vi "FBProjectVI.vi"(11 "Element":dbl=8.0) -> (0 "Element Index":dbl=3.0, 3 "Element Found":bool=TRUE)   [LabVIEW 2023]
doc: "Array = {5,3,8,9,1}\nOutput = Index of element"
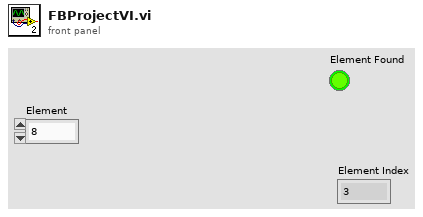
[diagram p1: front panel]
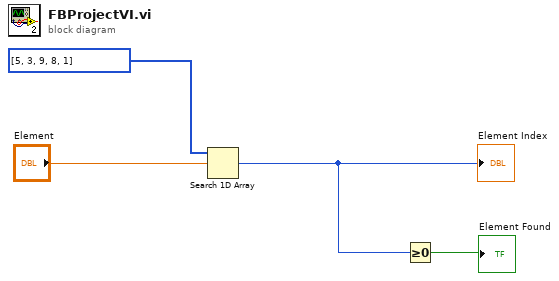
[diagram p0: block diagram]
diagram:
  n1 = Search 1D Array(1D array=i32[] [5, 3, 9, 8, 1], element="Element") -> (index of element=w2:i32)  [unwired: 1 in]
  "Element Index" <- w2
  n2 = Greater Or Equal To 0?(x=w2) -> (x >= 0?=→"Element Found":bool)
